vi "00EE.vi"(11 "Variables and Memory in":T1 {"GFX" format="%02x"}) -> (3 "Variables and Memory out":T1 {"GFX" format="%02x"})   [LabVIEW 2021]
uses:
  Controls/ClusterF.ctl
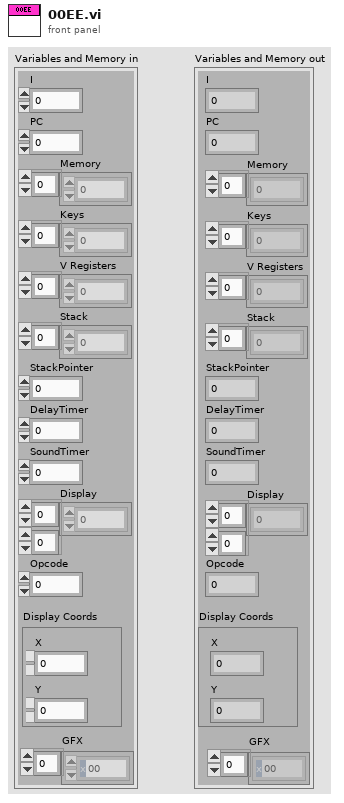
[diagram p1: front panel]
types:
  T1 = typedef "ClusterF.ctl" = cluster{"I":u16, "PC":u16, "Memory":u8[], "Keys":u8[], "V Registers":u8[], "Stack":u16[], "StackPointer":u16, "DelayTimer":u8, "SoundTimer":u8, "Display":u8[][], "Opcode":u16, "Display Coords":cluster{"X":u8, "Y":u8}, "GFX":u8[]}
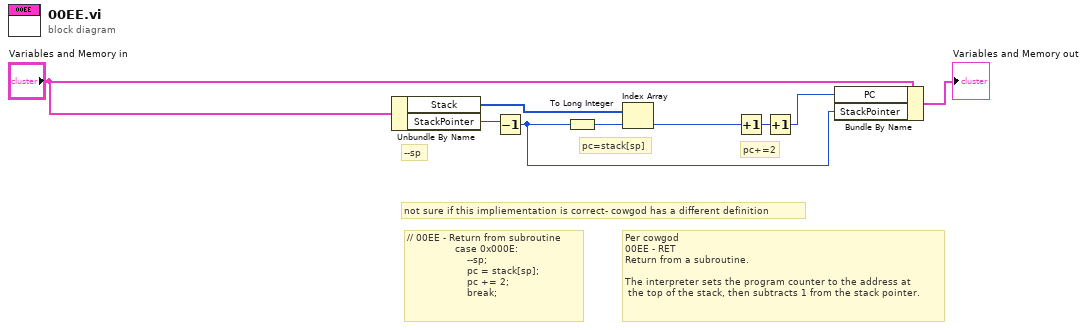
[diagram p0: block diagram]
diagram:
  # "Per cowgod\n00EE - RET\nReturn from a subroutine.\n\nThe interpreter sets the program counter to the address at\n the top of the stack, then subtracts 1 from the stack pointer."
  # "// 00EE - Return from subroutine\n                case 0x000E:\n                    --sp;\n                    pc = stack[sp];\n                    pc += 2;\n                    break;"
  # "not sure if this impliementation is correct- cowgod has a different definition"
  # "pc+=2"
  # "pc=stack[sp]"
  # "--sp"
  n1 = Unbundle By Name("Variables and Memory in") -> ("Stack"=w2:u16[], "StackPointer"=w1:u16)
  n2 = Decrement(x=w1) -> (x-1=w9:u16)
  n3 = To Long Integer(number=w9) -> (32bit integer=w8:i32)
  n4 = Index Array(array=w2, index=w8) -> (element=w4:u16)
  n5 = Increment(x=w4) -> (x+1=w3:u16)
  n6 = Increment(x=w3) -> (x+1=w7:u16)
  n7 = Bundle By Name(cluster="Variables and Memory in", "PC"=w7, "StackPointer"=w9) -> (→"Variables and Memory out":T1)
